vi "Open Control Key Down Filter Reference.vi"(8 "error in (no error)":errorcluster, 11 "IControlKeyDownFilter in":refnum<class "IControlKeyDownFilter.lvclass">) -> (0 "error out":errorcluster, 3 "ControlKeyDownFilter Reference":T1)   [LabVIEW 2015, in "ActorEvents.lvlib" / "IControlKeyDownFilter.lvclass"]
uses:
  IControlKeyDownFilter.lvclass
  ControlKeyDownFilter Reference.ctl
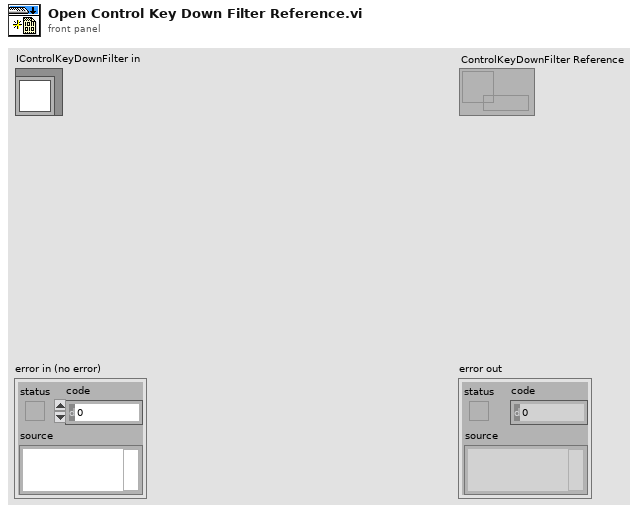
[diagram p1: front panel]
types:
  T1 = typedef "ActorEvents.lvlib/IControlKeyDownFilter.lvclass/ControlKeyDownFilter Reference.ctl" = refnum<data-value>
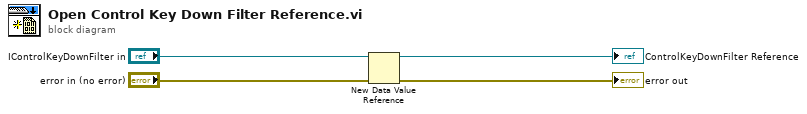
[diagram p0: block diagram]
diagram:
  n1 = New Data Value Reference(data value="IControlKeyDownFilter in", error in="error in (no error)") -> (data value reference=→"ControlKeyDownFilter Reference":refnum<data-value>, error out=→"error out":errorcluster)
